vi "CSTK_Button_Icon_get_ButtonSize.vi"(4 "error in (no error)":errorcluster caption="错误输入（无错误）", 6 "Container State":T19 caption="容器状态", 7 "Display State In":T1={"ButtonSize"={"False"={"Width"=0, "Height"=0}, "True"={"Width"=0, "Height"=0}, "True to False"={"Width"=0, "Height"=0}, "False to True"={"Width"=0, "Height"=0}, "Hover in False"={"Width"=0, "Height"=0}, "Hover in True"={"Width"=0, "Height"=0}}, "Logo Image"={"False"={"image type"=0, "image depth"=0, "image"=[], "mask"=[], "colors"=[], "Rectangle"={"left"=0, "top"=0, "right"=0, "bottom"=0}}, "True"={"image type"=0, "image depth"=0, "image"=[], "mask"=[], "colors"=[], "Rectangle"={"left"=0, "top"=0, "right"=0, "bottom"=0}}, "True to False"={"image type"=0, "image depth"=0, "image"=[], "mask"=[], "colors"=[], "Rectangle"={"left"=0, "top"=0, "right"=0, "bottom"=0}}, "False to True"={"image type"=0, "image depth"=0, "image"=[], "mask"=[], "colors"=[], "Rectangle"={"left"=0, "top"=0, "right"=0, "bottom"=0}}, "Hover in False"={"image type"=0, "image depth"=0, "image"=[], "mask"=[], "colors"=[], "Rectangle"={"left"=0, "top"=0, "right"=0, "bottom"=0}}, "Hover in True"={"image type"=0, "image depth"=0, "image"=[], "mask"=[], "colors"=[], "Rectangle"={"left"=0, "top"=0, "right"=0, "bottom"=0}}}, "Logo Properties"={"False"={"Display Logo?"=FALSE, "Horizontal Offset"=0}, "True"={"Display Logo?"=FALSE, "Horizontal Offset"=0}, "True to False"={"Display Logo?"=FALSE, "Horizontal Offset"=0}, "False to True"={"Display Logo?"=FALSE, "Horizontal Offset"=0}, "Hover in False"={"Display Logo?"=FALSE, "Horizontal Offset"=0}, "Hover in True"={"Display Logo?"=FALSE, "Horizontal Offset"=0}}, "Text String"={"False"="", "True"="", "True to False"="", "False to True"="", "Hover in False"="", "Hover in True"=""}, "Text Properties"={"False"={"Display Text?"=FALSE, "Text Color"=0, "Horizontal Offset"=0, "Font Style"={"Font Name"="", "Size"=0, "Strikeout?"=FALSE, "Italic?"=FALSE, "Underline?"=FALSE, "Outline?"=FALSE, "Shadow?"=FALSE, "Bold?"=FALSE}}, "True"={"Display Text?"=FALSE, "Text Color"=0, "Horizontal Offset"=0, "Font Style"={"Font Name"="", "Size"=0, "Strikeout?"=FALSE, "Italic?"=FALSE, "Underline?"=FALSE, "Outline?"=FALSE, "Shadow?"=FALSE, "Bold?"=FALSE}}, "True to False"={"Display Text?"=FALSE, "Text Color"=0, "Horizontal Offset"=0, "Font Style"={"Font Name"="", "Size"=0, "Strikeout?"=FALSE, "Italic?"=FALSE, "Underline?"=FALSE, "Outline?"=FALSE, "Shadow?"=FALSE, "Bold?"=FALSE}}, "False to True"={"Display Text?"=FALSE, "Text Color"=0, "Horizontal Offset"=0, "Font Style"={"Font Name"="", "Size"=0, "Strikeout?"=FALSE, "Italic?"=FALSE, "Underline?"=FALSE, "Outline?"=FALSE, "Shadow?"=FALSE, "Bold?"=FALSE}}, "Hover in False"={"Display Text?"=FALSE, "Text Color"=0, "Horizontal Offset"=0, "Font Style"={"Font Name"="", "Size"=0, "Strikeout?"=FALSE, "Italic?"=FALSE, "Underline?"=FALSE, "Outline?"=FALSE, "Shadow?"=FALSE, "Bold?"=FALSE}}, "Hover in True"={"Display Text?"=FALSE, "Text Color"=0, "Horizontal Offset"=0, "Font Style"={"Font Name"="", "Size"=0, "Strikeout?"=FALSE, "Italic?"=FALSE, "Underline?"=FALSE, "Outline?"=FALSE, "Shadow?"=FALSE, "Bold?"=FALSE}}}, "BG Color"={"False"=0, "True"=0, "True to False"=0, "False to True"=0, "Hover in False"=0, "Hover in True"=0}, "Border Color"={"False"=0, "True"=0, "True to False"=0, "False to True"=0, "Hover in False"=0, "Hover in True"=0}, "Border Properties"={"False"={"Radius"=0, "Border Style"={"Width"=3, "Style"=enum."Solid"}}, "True"={"Radius"=0, "Border Style"={"Width"=3, "Style"=enum."Solid"}}, "True to False"={"Radius"=0, "Border Style"={"Width"=3, "Style"=enum."Solid"}}, "False to True"={"Radius"=0, "Border Style"={"Width"=3, "Style"=enum."Solid"}}, "Hover in False"={"Radius"=0, "Border Style"={"Width"=3, "Style"=enum."Solid"}}, "Hover in True"={"Radius"=0, "Border Style"={"Width"=3, "Style"=enum."Solid"}}}, "Current BG Image"={"False"=bytes[0], "True"=bytes[0], "True to False"=bytes[0], "False to True"=bytes[0], "Hover in False"=bytes[0], "Hover in True"=bytes[0]}, "DrawAreaSize"={"False"={"Width"=0, "Height"=0}, "True"={"Width"=0, "Height"=0}, "True to False"={"Width"=0, "Height"=0}, "False to True"={"Width"=0, "Height"=0}, "Hover in False"={"Width"=0, "Height"=0}, "Hover in True"={"Width"=0, "Height"=0}}, "Text String Offset"={"False"=0, "True"=0, "True to False"=0, "False to True"=0, "Hover in False"=0, "Hover in True"=0}} caption="显示状态输入") -> (0 "error out":errorcluster caption="错误输出", 2 "Value":T3 caption="值", 3 "Display State Out":T1={"ButtonSize"={"False"={"Width"=0, "Height"=0}, "True"={"Width"=0, "Height"=0}, "True to False"={"Width"=0, "Height"=0}, "False to True"={"Width"=0, "Height"=0}, "Hover in False"={"Width"=0, "Height"=0}, "Hover in True"={"Width"=0, "Height"=0}}, "Logo Image"={"False"={"image type"=0, "image depth"=0, "image"=[], "mask"=[], "colors"=[], "Rectangle"={"left"=0, "top"=0, "right"=0, "bottom"=0}}, "True"={"image type"=0, "image depth"=0, "image"=[], "mask"=[], "colors"=[], "Rectangle"={"left"=0, "top"=0, "right"=0, "bottom"=0}}, "True to False"={"image type"=0, "image depth"=0, "image"=[], "mask"=[], "colors"=[], "Rectangle"={"left"=0, "top"=0, "right"=0, "bottom"=0}}, "False to True"={"image type"=0, "image depth"=0, "image"=[], "mask"=[], "colors"=[], "Rectangle"={"left"=0, "top"=0, "right"=0, "bottom"=0}}, "Hover in False"={"image type"=0, "image depth"=0, "image"=[], "mask"=[], "colors"=[], "Rectangle"={"left"=0, "top"=0, "right"=0, "bottom"=0}}, "Hover in True"={"image type"=0, "image depth"=0, "image"=[], "mask"=[], "colors"=[], "Rectangle"={"left"=0, "top"=0, "right"=0, "bottom"=0}}}, "Logo Properties"={"False"={"Display Logo?"=FALSE, "Horizontal Offset"=0}, "True"={"Display Logo?"=FALSE, "Horizontal Offset"=0}, "True to False"={"Display Logo?"=FALSE, "Horizontal Offset"=0}, "False to True"={"Display Logo?"=FALSE, "Horizontal Offset"=0}, "Hover in False"={"Display Logo?"=FALSE, "Horizontal Offset"=0}, "Hover in True"={"Display Logo?"=FALSE, "Horizontal Offset"=0}}, "Text String"={"False"="", "True"="", "True to False"="", "False to True"="", "Hover in False"="", "Hover in True"=""}, "Text Properties"={"False"={"Display Text?"=FALSE, "Text Color"=0, "Horizontal Offset"=0, "Font Style"={"Font Name"="", "Size"=0, "Strikeout?"=FALSE, "Italic?"=FALSE, "Underline?"=FALSE, "Outline?"=FALSE, "Shadow?"=FALSE, "Bold?"=FALSE}}, "True"={"Display Text?"=FALSE, "Text Color"=0, "Horizontal Offset"=0, "Font Style"={"Font Name"="", "Size"=0, "Strikeout?"=FALSE, "Italic?"=FALSE, "Underline?"=FALSE, "Outline?"=FALSE, "Shadow?"=FALSE, "Bold?"=FALSE}}, "True to False"={"Display Text?"=FALSE, "Text Color"=0, "Horizontal Offset"=0, "Font Style"={"Font Name"="", "Size"=0, "Strikeout?"=FALSE, "Italic?"=FALSE, "Underline?"=FALSE, "Outline?"=FALSE, "Shadow?"=FALSE, "Bold?"=FALSE}}, "False to True"={"Display Text?"=FALSE, "Text Color"=0, "Horizontal Offset"=0, "Font Style"={"Font Name"="", "Size"=0, "Strikeout?"=FALSE, "Italic?"=FALSE, "Underline?"=FALSE, "Outline?"=FALSE, "Shadow?"=FALSE, "Bold?"=FALSE}}, "Hover in False"={"Display Text?"=FALSE, "Text Color"=0, "Horizontal Offset"=0, "Font Style"={"Font Name"="", "Size"=0, "Strikeout?"=FALSE, "Italic?"=FALSE, "Underline?"=FALSE, "Outline?"=FALSE, "Shadow?"=FALSE, "Bold?"=FALSE}}, "Hover in True"={"Display Text?"=FALSE, "Text Color"=0, "Horizontal Offset"=0, "Font Style"={"Font Name"="", "Size"=0, "Strikeout?"=FALSE, "Italic?"=FALSE, "Underline?"=FALSE, "Outline?"=FALSE, "Shadow?"=FALSE, "Bold?"=FALSE}}}, "BG Color"={"False"=0, "True"=0, "True to False"=0, "False to True"=0, "Hover in False"=0, "Hover in True"=0}, "Border Color"={"False"=0, "True"=0, "True to False"=0, "False to True"=0, "Hover in False"=0, "Hover in True"=0}, "Border Properties"={"False"={"Radius"=0, "Border Style"={"Width"=3, "Style"=enum."Solid"}}, "True"={"Radius"=0, "Border Style"={"Width"=3, "Style"=enum."Solid"}}, "True to False"={"Radius"=0, "Border Style"={"Width"=3, "Style"=enum."Solid"}}, "False to True"={"Radius"=0, "Border Style"={"Width"=3, "Style"=enum."Solid"}}, "Hover in False"={"Radius"=0, "Border Style"={"Width"=3, "Style"=enum."Solid"}}, "Hover in True"={"Radius"=0, "Border Style"={"Width"=3, "Style"=enum."Solid"}}}, "Current BG Image"={"False"=bytes[0], "True"=bytes[0], "True to False"=bytes[0], "False to True"=bytes[0], "Hover in False"=bytes[0], "Hover in True"=bytes[0]}, "DrawAreaSize"={"False"={"Width"=0, "Height"=0}, "True"={"Width"=0, "Height"=0}, "True to False"={"Width"=0, "Height"=0}, "False to True"={"Width"=0, "Height"=0}, "Hover in False"={"Width"=0, "Height"=0}, "Hover in True"={"Width"=0, "Height"=0}}, "Text String Offset"={"False"=0, "True"=0, "True to False"=0, "False to True"=0, "Hover in False"=0, "Hover in True"=0}} caption="显示状态输出")   [LabVIEW 2015, in "CSTK_Button_Icon.xctl"]
uses:
  CSTK_Button_Icon.xctl
  <vilib>/_xctls/Container State.ctl
  <vilib>/Utility/miscctls.llb/LVBoundsTypeDef.ctl
  CSTK_Button_Icon_Status.ctl
  Private/TypeDefinitions/_CSTK_Button_Icon_ButtonSize.ctl
  Private/TypeDefinitions/_CSTK_Button_Icon_LogoImage.ctl
  <vilib>/picture/picture.llb/imagedata.ctl
  Private/TypeDefinitions/_CSTK_Button_Icon_LogoProperties.ctl
  Private/TypeDefinitions/_CSTK_Button_Icon_LogoProperties_Data.ctl
  Private/TypeDefinitions/_CSTK_Button_Icon_TextString.ctl
  Private/TypeDefinitions/_CSTK_Button_Icon_TextProperties.ctl
  Private/TypeDefinitions/_CSTK_Button_Icon_TextProperties_Data.ctl
  Private/TypeDefinitions/_CSTK_Button_Icon_TextProperties_FontStyle.ctl
  Private/TypeDefinitions/_CSTK_Button_Icon_BGColor.ctl
  Private/TypeDefinitions/_CSTK_Button_Icon_BorderColor.ctl
  Private/TypeDefinitions/_CSTK_Button_Icon_BorderProperties.ctl
  Private/TypeDefinitions/_CSTK_Button_Icon_BorderProperties_Data.ctl
  Private/TypeDefinitions/_CSTK_Button_Icon_CurrentBGImage.ctl
  Private/TypeDefinitions/_CSTK_Button_Icon_DrawAreaSize.ctl
  Private/TypeDefinitions/_CSTK_Button_Icon_TextStartOffset.ctl
  <vilib>/_xctls/XControlSupport.lvlib
panel:
  # "将以下值显示控件替换为所需类型的显示控件。\n不要从连线板中删除该显示控件或其它显示控件。\n不要更改连线板模式。\n值显示控件应始终位于连线板输出端自顶部起第二个接线端。"
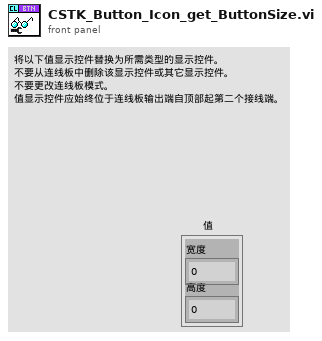
[diagram p1: front panel]
types:
  T1 = typedef "CSTK_Button_Icon.xctl/CSTK_Button_Icon_Status.ctl" = cluster{"ButtonSize":T2, "Logo Image":T4, "Logo Properties":T6, "Text String":T8, "Text Properties":T9, "BG Color":T12, "Border Color":T13, "Border Properties":T14, "Current BG Image":T16, "DrawAreaSize":T17, "Text String Offset":T18}
  T2 = typedef "CSTK_Button_Icon.xctl/_CSTK_Button_Icon_ButtonSize.ctl" = cluster{"False":T3, "True":T3, "True to False":T3, "False to True":T3, "Hover in False":T3, "Hover in True":T3}
  T3 = typedef "LVBoundsTypeDef.ctl" = cluster{"Width":u32, "Height":u32}
  T4 = typedef "CSTK_Button_Icon.xctl/_CSTK_Button_Icon_LogoImage.ctl" = cluster{"False":T5, "True":T5, "True to False":T5, "False to True":T5, "Hover in False":T5, "Hover in True":T5}
  T5 = typedef "imagedata.ctl" = cluster{"image type":i32, "image depth":i32, "image":u8[], "mask":u8[], "colors":u32[], "Rectangle":cluster{"left":i16, "top":i16, "right":i16, "bottom":i16}}
  T6 = typedef "CSTK_Button_Icon.xctl/_CSTK_Button_Icon_LogoProperties.ctl" = cluster{"False":T7, "True":T7, "True to False":T7, "False to True":T7, "Hover in False":T7, "Hover in True":T7}
  T7 = typedef "CSTK_Button_Icon.xctl/_CSTK_Button_Icon_LogoProperties_Data.ctl" = cluster{"Display Logo?":bool, "Horizontal Offset":i16}
  T8 = typedef "CSTK_Button_Icon.xctl/_CSTK_Button_Icon_TextString.ctl" = cluster{"False":string, "True":string, "True to False":string, "False to True":string, "Hover in False":string, "Hover in True":string}
  T9 = typedef "CSTK_Button_Icon.xctl/_CSTK_Button_Icon_TextProperties.ctl" = cluster{"False":T10, "True":T10, "True to False":T10, "False to True":T10, "Hover in False":T10, "Hover in True":T10}
  T10 = typedef "CSTK_Button_Icon.xctl/_CSTK_Button_Icon_TextProperties_Data.ctl" = cluster{"Display Text?":bool, "Text Color":u32, "Horizontal Offset":i16, "Font Style":T11}
  T11 = typedef "CSTK_Button_Icon.xctl/_CSTK_Button_Icon_TextProperties_FontStyle.ctl" = cluster{"Font Name":string, "Size":i16, "Strikeout?":bool, "Italic?":bool, "Underline?":bool, "Outline?":bool, "Shadow?":bool, "Bold?":bool}
  T12 = typedef "CSTK_Button_Icon.xctl/_CSTK_Button_Icon_BGColor.ctl" = cluster{"False":u32, "True":u32, "True to False":u32, "False to True":u32, "Hover in False":u32, "Hover in True":u32}
  T13 = typedef "CSTK_Button_Icon.xctl/_CSTK_Button_Icon_BorderColor.ctl" = cluster{"False":u32, "True":u32, "True to False":u32, "False to True":u32, "Hover in False":u32, "Hover in True":u32}
  T14 = typedef "CSTK_Button_Icon.xctl/_CSTK_Button_Icon_BorderProperties.ctl" = cluster{"False":T15, "True":T15, "True to False":T15, "False to True":T15, "Hover in False":T15, "Hover in True":T15}
  T15 = typedef "CSTK_Button_Icon.xctl/_CSTK_Button_Icon_BorderProperties_Data.ctl" = cluster{"Radius":i16, "Border Style":cluster{"Width":u16, "Style":enum32{"Solid", "Dash", "Dot", "DashDot", "DashDotDot"}}}
  T16 = typedef "CSTK_Button_Icon.xctl/_CSTK_Button_Icon_CurrentBGImage.ctl" = cluster{"False":picture, "True":picture, "True to False":picture, "False to True":picture, "Hover in False":picture, "Hover in True":picture}
  T17 = typedef "CSTK_Button_Icon.xctl/_CSTK_Button_Icon_DrawAreaSize.ctl" = cluster{"False":T3, "True":T3, "True to False":T3, "False to True":T3, "Hover in False":T3, "Hover in True":T3}
  T18 = typedef "CSTK_Button_Icon.xctl/_CSTK_Button_Icon_TextStartOffset.ctl" = cluster{"False":i32, "True":i32, "True to False":i32, "False to True":i32, "Hover in False":i32, "Hover in True":i32}
  T19 = typedef "XControlSupport.lvlib/Container State.ctl" = cluster{"Indicator?":bool, "Run Mode?":bool, " Refnum":refnum<vi>}
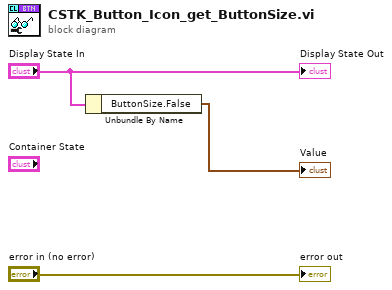
[diagram p0: block diagram]
diagram:
  n1 = Unbundle By Name("Display State In") -> ("ButtonSize.False"=→"Value":T3)
  "error out" <- "error in (no error)"
  "Display State Out" <- "Display State In"
